vi "select_roi.vi"(8 "error in (no error)":errorcluster, 10 "path in":path, 11 "TrajectoryMH100122AODRAPS in":refnum<class "TrajectoryMH100122AODRAPS.lvclass">) -> (0 "error out":errorcluster, 2 "selected path out":path, 3 "TrajectoryMH100122AODRAPS out":refnum<class "TrajectoryMH100122AODRAPS.lvclass">)   [LabVIEW 2010, in "TrajectoryMH100122AODRAPS.lvclass"]
uses:
  TrajectoryMH100122AODRAPS.lvclass
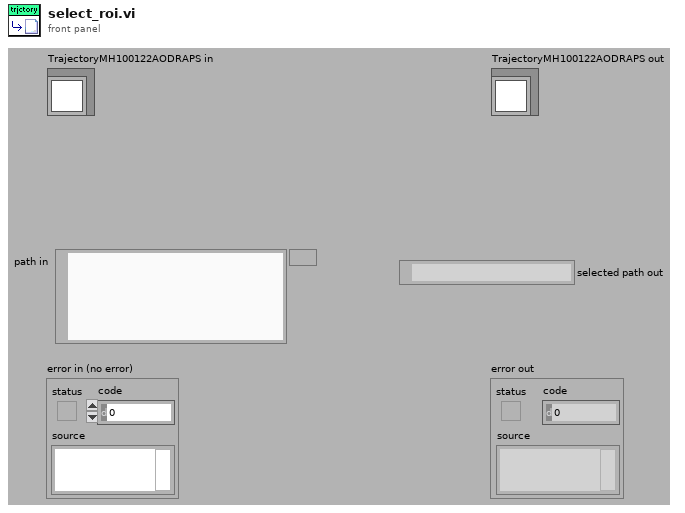
[diagram p1: front panel]
types:
  T1 = cluster{"Creation Time (string)":string, "Last Access Time (string)":string, "Last Write Time (string)":string}
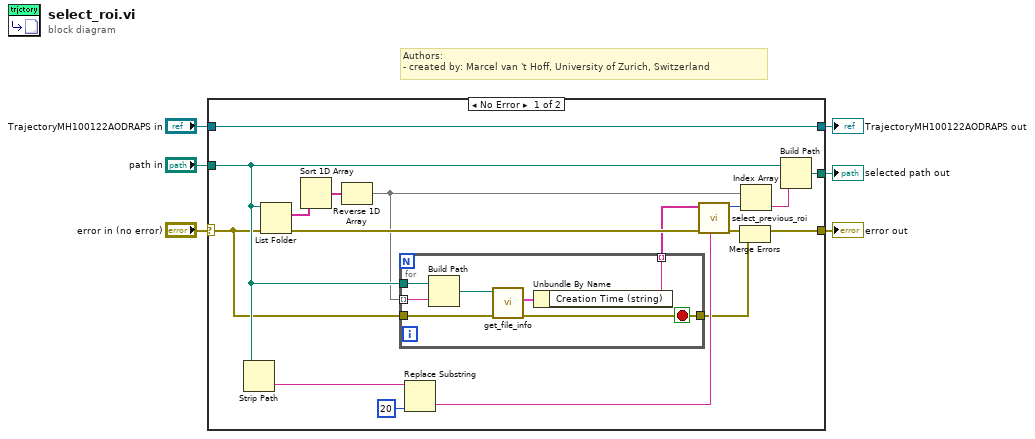
[diagram p0: block diagram]
diagram:
  # "Authors: \n- created by: Marcel van 't Hoff, University of Zurich, Switzerland"
  n1 = case shown="No Error" "error in (no error)" {
    selector: "error in (no error)" -> [w13 w32]
    tunnel: [w12 w32] -> w5
    tunnel: [w23 w31] -> w3
    tunnel: "TrajectoryMH100122AODRAPS in" -> [w23 w31]
    tunnel: "path in" -> [w14 _]
    tunnel: [w15 _] -> w1
    frame No Error {
      n2 = Strip Path(path=w14) -> (name=w20:string)  [unwired: 1 out]
      n3 = List Folder(path=w14, error in=w13) -> (filenames=w8:string[], error out=w22:errorcluster)  [unwired: 2 in, 2 out]
      n4 = Sort 1D Array(array=w8) -> (sorted array=w9:string[])
      n5 = Reverse 1D Array(array=w9) -> (reversed array=w7:string[])
      n6 = for {
        tunnel: w7 -> [w29] mode=indexing
        tunnel: [w28] -> w10 mode=indexing
        tunnel: w14 -> [w30]
        tunnel: w13 -> [w27]
        tunnel: [w25] -> w11
        stop <- w25 stop-if-true
        n7 = Build Path(base path=w30, name or relative path=w29) -> (appended path=w26:path)
        n8 = call "get_file_info.vi"("error in (no error)"=w27, "File Path in"=w26) -> ("error out"=w25:errorcluster, "String Times"=w24:T1)  [unwired: 7 in, 1 out]
        n9 = Unbundle By Name(w24) -> ("Creation Time (string)"=w28:string)
      }
      n10 = Replace Substring(2:20 ("length (len. of substring)"), 5:w20) -> (0:w18:string)  [unwired: 2 in, 1 out]
      n11 = call "select_previous_roi.vi"("title in"=w18, "error in"=w22, "times in"=w10) -> ("error out"=w21:errorcluster, "selector out"=w17:i32)  [unwired: 7 in]
      n12 = Merge Errors(w21, w11) -> (w12:errorcluster)
      n13 = Index Array(array=w7, index=w17) -> (element=w16:string)
      n14 = Build Path(base path=w14, name or relative path=w16) -> (appended path=w15:path)
    }
    frame Error {
    }
  }
  "error out" <- w5
  "TrajectoryMH100122AODRAPS out" <- w3
  "selected path out" <- w1
